vi "show_all_Fotos_B.vi"() -> ()   [LabVIEW 2017]
panel:
  in  "foto#":dbl(slide)=1.0 scale=0.0..121.0
  out "Tot.#Fotos":i32
  out "Boolean Round":bool
  in  "Power On Button":bool
  out "idx":i32
  out "imagePath":path
  in  "Folder":path=path "C:/Imagenes/experimentos"
  out "Resized Picture":picture
  # "Lector de imágenes"
  # "asslcdms Feb2023 LV17"
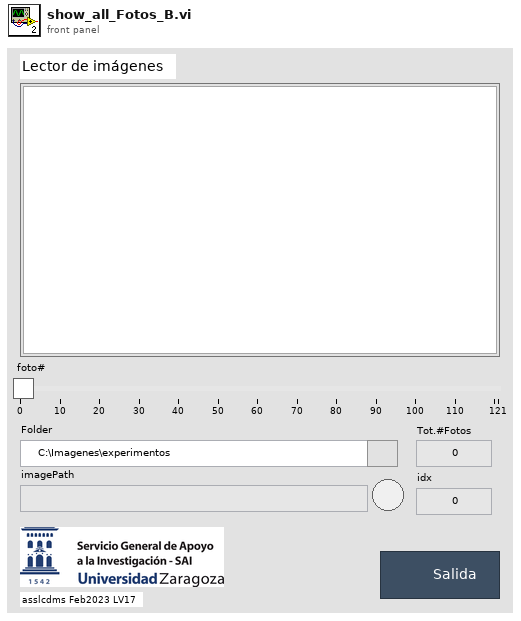
[diagram p1: front panel]
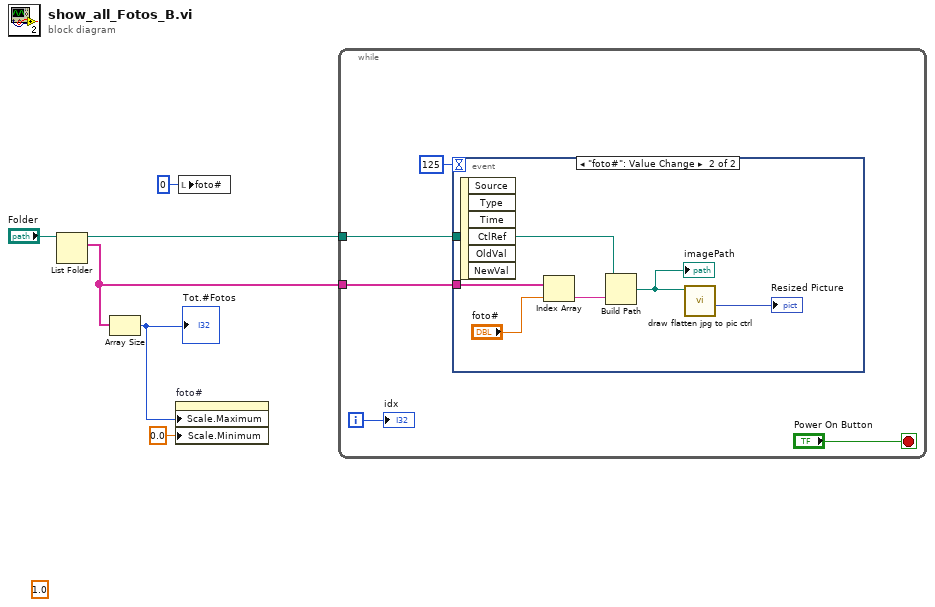
[diagram p0: block diagram]
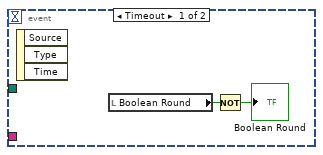
[diagram p2: hidden frame]
diagram:
  (unwired) 1.0 ("Horizontal Slider Control")
  n1 = List Folder(path="Folder") -> (path out=w5:path, filenames=w4:string[])  [unwired: 3 in, 2 out]
  n2 = Array Size(array=w4) -> (size(s)=w3:i32)
  "Tot.#Fotos" <- w3
  n3 = property on="foto#" class="Slide (strict)"("Scale.Maximum"=w3, "Scale.Minimum"=0.0 ("Scale.Range:Minimum")) -> ()  [unwired: 2 in, 2 out]
  n4 = local write "foto#"(0 ("foto#")) -> ()
  n5 = while {
    tunnel: w5 -> [w11]
    tunnel: w4 -> [w8]
    i -> [w10]
    stop <- "Power On Button" stop-if-true
    n6 = event shown="[1] \"foto#\": Value Change" {
      selector: _ -> [_ _]
      dyn-events: _ -> [_ _]
      timeout: 125 -> [_ _]
      tunnel: w11 -> [_ w15]
      tunnel: w8 -> [_ w16]
      event Timeout {
        n7 = event-data() -> ()  [unwired: 1 in, 3 out]
        n8 = local read "Boolean Round"() -> (w12:bool)
        n9 = Not(x=w12) -> (.not. x?=→"Boolean Round":bool)
      }
      event "foto#": Value Change {
        n10 = event-data() -> ()  [unwired: 1 in, 6 out]
        n11 = Index Array(array=w16, index="foto#") -> (element=w17:string)
        n12 = Build Path(base path=w15, name or relative path=w17) -> (appended path=w19:path)
        "imagePath" <- w19
        n13 = call "draw flatten jpg to pic ctrl.vi"("path to JPEG file"=w19) -> ("Picture"=→"Resized Picture":picture)  [unwired: 9 in, 1 out]
      }
    }
    "idx" <- w10
  }
